vi "Contex Menu Selection.vi"(8 "error in (no error)":errorcluster, 10 "MenuItem":string, 11 "HIJ Vision File Viewer in":refnum<class "HIJ Vision File Display.lvclass">) -> (0 "error out":errorcluster, 3 "HIJ Vision File Viewer out":refnum<class "HIJ Vision File Display.lvclass">)   [LabVIEW 2014, in "HIJ Vision File Display.lvlib" / "HIJ Vision File Display.lvclass"]
uses:
  HIJ Vision File Display.lvclass
  HIJ Vision File Display.lvclass/HIJ Vision File Display.ctl
  Display Actors/HIJ Vision Display/HIJ Vision Display/HIJ Vision Display.lvclass
  <vilib>/Utility/config.llb/NI_LVConfig.lvlib
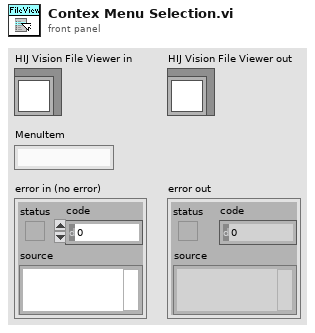
[diagram p1: front panel]
types:
  T1 = typedef "NI_LVConfig.lvlib/Config Data RefNum.ctl" = refnum<k1>
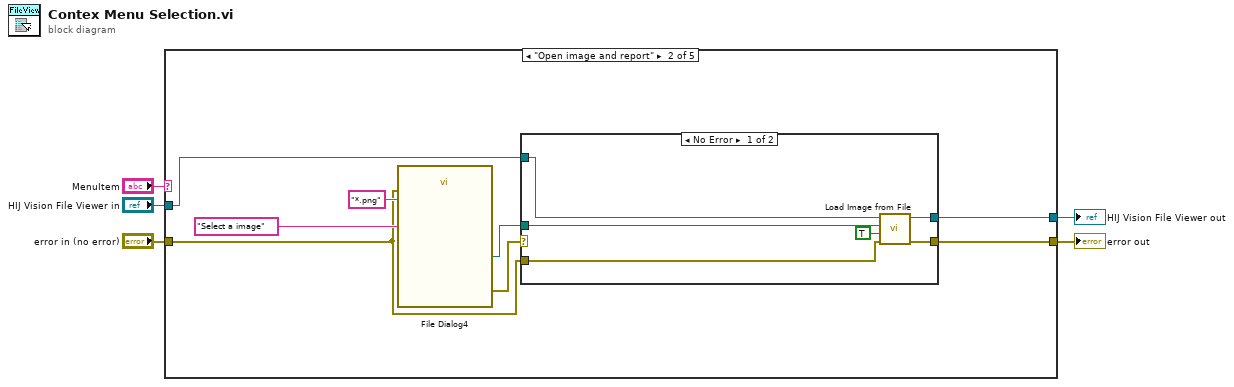
[diagram p0: block diagram]
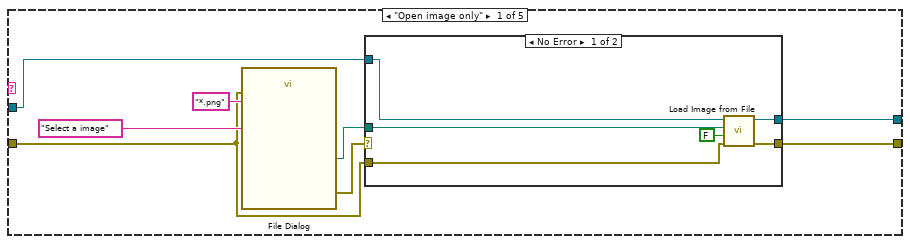
[diagram p2: hidden frame]
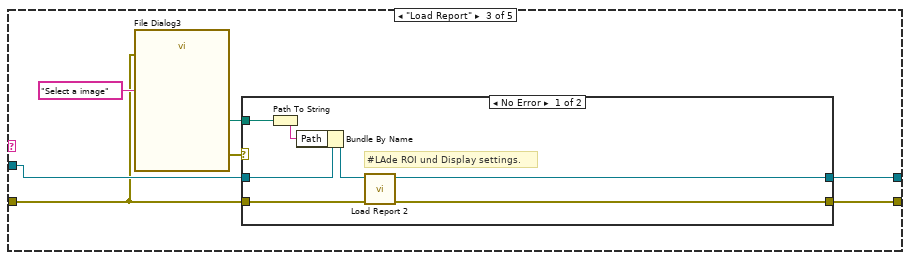
[diagram p5: hidden frame]
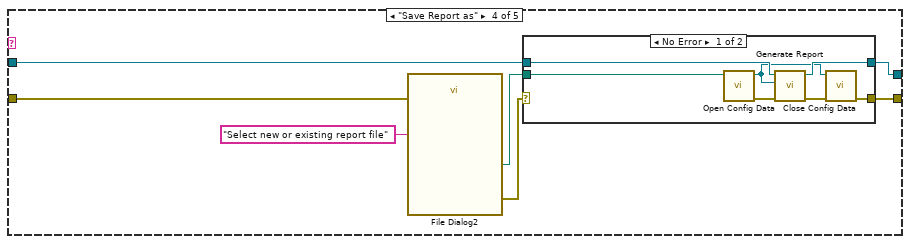
[diagram p7: hidden frame]
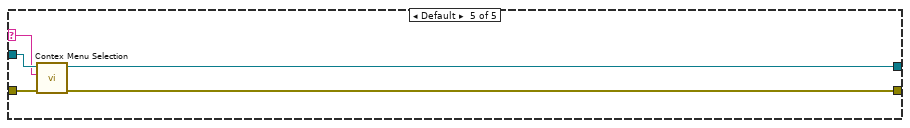
[diagram p9: hidden frame]
diagram:
  n1 = case shown="\"Open image and report\"" "MenuItem" {
    selector: "MenuItem" -> [_ _ _ _ w70]
    tunnel: [w8 w24 w40 w55 w74] -> w5
    tunnel: [w9 w25 w41 w56 w73] -> w4
    tunnel: "error in (no error)" -> [w6 w22 w38 w60 w72]
    tunnel: "HIJ Vision File Viewer in" -> [w11 w27 w43 w58 w71]
    frame "Open image only" {
      n2 = call "File Dialog"("prompt"="Select a image", "error in"=w6, "pattern (all files)"="*.png") -> ("selected path"=w10:path, "error out"=w7:errorcluster)  [unwired: 9 in, 2 out]
      n3 = case shown="No Error" w7 {
        tunnel: w11 -> [w19 w21]
        tunnel: w6 -> [w16 w20]
        tunnel: w10 -> [w15 _]
        tunnel: [w18 w21] -> w9
        tunnel: [w17 w20] -> w8
        frame No Error {
          n4 = call-dynamic "Load Image from File.vi"("error in (no error)"=w16, "Load Report"=FALSE, "Image"=w15, "HIJ Vision File Viewer in"=w19) -> ("error out"=w17:errorcluster, "HIJ Vision File Viewer out"=w18:refnum<class "HIJ Vision File Display.lvclass">)  [unwired: 6 in]
        }
        frame Error {
        }
      }
    }
    frame "Open image and report" {
      n5 = call "File Dialog4"("prompt"="Select a image", "error in"=w22, "pattern (all files)"="*.png") -> ("selected path"=w26:path, "error out"=w23:errorcluster)  [unwired: 9 in, 2 out]
      n6 = case shown="No Error" w23 {
        tunnel: w27 -> [w35 w37]
        tunnel: w22 -> [w32 w36]
        tunnel: w26 -> [w31 _]
        tunnel: [w34 w37] -> w25
        tunnel: [w33 w36] -> w24
        frame No Error {
          n7 = call-dynamic "Load Image from File.vi"("error in (no error)"=w32, "Load Report"=TRUE, "Image"=w31, "HIJ Vision File Viewer in"=w35) -> ("error out"=w33:errorcluster, "HIJ Vision File Viewer out"=w34:refnum<class "HIJ Vision File Display.lvclass">)  [unwired: 6 in]
        }
        frame Error {
        }
      }
    }
    frame "Load Report" {
      n8 = call "File Dialog3"("prompt"="Select a image", "error in"=w38) -> ("selected path"=w42:path, "error out"=w39:errorcluster)  [unwired: 10 in, 2 out]
      n9 = case shown="No Error" w39 {
        tunnel: w43 -> [w51 w53]
        tunnel: w42 -> [w46 _]
        tunnel: [w50 w53] -> w41
        tunnel: [w49 w52] -> w40
        tunnel: w38 -> [w48 w52]
        frame No Error {
          # "#LAde ROI und Display settings."
          n10 = Path To String(path=w46) -> (string=w45:string)
          n11 = Bundle By Name(cluster=w51, "Path"=w45) -> (w47:refnum<class "HIJ Vision File Display.lvclass">)
          n12 = call-dynamic "Load Report 2.vi"("error in (no error)"=w48, "HIJ Vision File Viewer in"=w47) -> ("error out"=w49:errorcluster, "HIJ Vision File Viewer out"=w50:refnum<class "HIJ Vision File Display.lvclass">)  [unwired: 8 in]
        }
        frame Error {
        }
      }
    }
    frame "Save Report as" {
      n13 = call "File Dialog2"("prompt"="Select new or existing report file", "error in"=w60) -> ("selected path"=w57:path, "error out"=w54:errorcluster)  [unwired: 10 in, 2 out]
      n14 = case shown="No Error" w54 {
        selector: w54 -> [_ w68]
        tunnel: w58 -> [w67 w69]
        tunnel: w57 -> [w64 _]
        tunnel: [w66 w69] -> w56
        tunnel: [w62 w68] -> w55
        frame No Error {
          n15 = call <vilib>:"Open Config Data.vi"("configuration file path"=w64) -> ("error out"=w63:errorcluster, "refnum"=w61:T1)  [unwired: 8 in, 1 out]
          n16 = call-dynamic "Generate Report.vi"("error in (no error)"=w63, "Resource In"=w61, "HIJ Vision File Viewer in"=w67) -> ("error out"=w65:errorcluster, "HIJ Vision File Viewer out"=w66:refnum<class "HIJ Vision File Display.lvclass">)  [unwired: 6 in, 1 out]
          n17 = call <vilib>:"Close Config Data.vi"("error in (no error)"=w65, "refnum"=w61) -> ("error out"=w62:errorcluster)  [unwired: 8 in, 1 out]
        }
        frame Error {
        }
      }
    }
    frame Default {
      n18 = call-parent "Contex Menu Selection.vi"("error in (no error)"=w72, "MenuItem"=w70, "HIJ Vision Display in"=w71) -> ("error out"=w74:errorcluster, "HIJ Vision Display out"=w73:refnum<class "HIJ Vision File Display.lvclass">)  [unwired: 7 in]
    }
  }
  "error out" <- w5
  "HIJ Vision File Viewer out" <- w4
